vi "Unicode String to Integer [ ].vi"(0 "Char U16 [ ] IN":u16[](array[numeric]), 2 "From":enum16{"String", "U16 [ ]"}(ring), 7 "Unicode String":string, 11 "error in (no error)":errorcluster) -> (4 "Unicode String OUT":string, 8 "Char U16 [ ]":u16[](array[numeric]), 15 "error duplicate":errorcluster)   [LabVIEW 2020, in "Exaprom PDF.lvlib"]
doc: "Version 1.1\nDeveloped by Jean-Marc Simard\nCopyright © 2012, Exaprom Inc.\nAll rights reserved.\nLicense: BSD\n\nWith iTextSharp 4.1.6 (http://itextsharp.sourceforge.net)\nunder Mozilla Public License Version 1.1\n(http://www.mozilla.org/MPL/MPL-1.1.html)"
uses:
  <userlib>/labview-PDF-writer-master/Exaprom PDF.lvlib
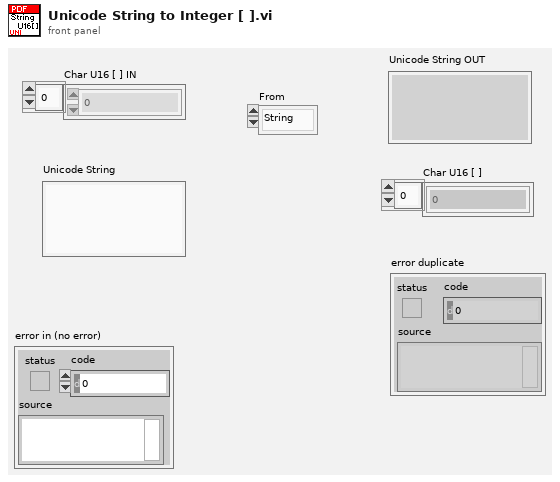
[diagram p1: front panel]
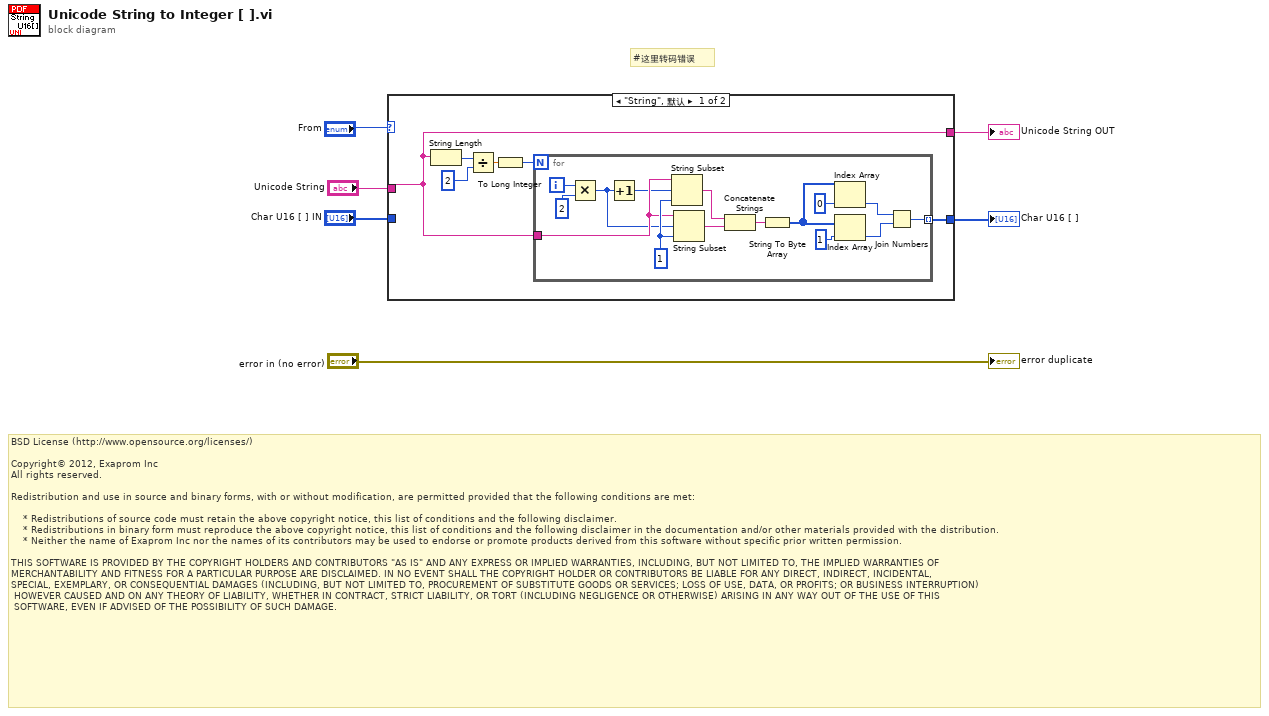
[diagram p0: block diagram]
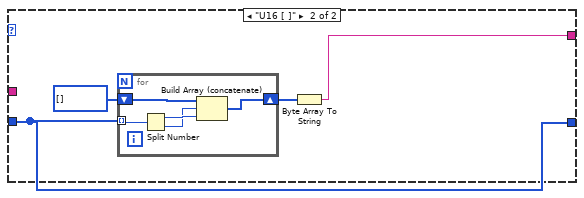
[diagram p2: hidden frame]
diagram:
  # "#这里转码错误"
  # "BSD License (http://www.opensource.org/licenses/)\n\nCopyright© 2012, Exaprom Inc\nAll rights reserved.\n\nRedistribution and use in source and binary forms, with or without modification, are permitted provided that the following conditions are met:\n\n    * Redistributions of source code must retain the above copyright notice, this list of conditions and the following disclaimer.\n    * Redistributions in binary form must reproduce the above copyright notice, this list of conditions and the following disclaimer in the documentation and/or other materials provided with the distribution.\n    * Neither the name of Exaprom Inc nor the names of its contributors may be used to endorse or promote products derived from this software without specific prior written permission.\n\nTHIS SOFTWARE IS PROVIDED BY THE COPYRIGHT HOLDERS AND CONTRIBUTORS \"AS IS\" AND ANY EXPRESS OR IMPLIED WARRANTIES, INCLUDING, BUT NOT LIMITED TO, THE IMPLIED WARRANTIES OF \nMERCHANTABILITY AND FITNESS FOR A PARTICULAR PURPOSE ARE DISCLAIMED. IN NO EVENT SHALL THE COPYRIGHT HOLDER OR CONTRIBUTORS BE LIABLE FOR ANY DIRECT, INDIRECT, INCIDENTAL,\nSPECIAL, EXEMPLARY, OR CONSEQUENTIAL DAMAGES (INCLUDING, BUT NOT LIMITED TO, PROCUREMENT OF SUBSTITUTE GOODS OR SERVICES; LOSS OF USE, DATA, OR PROFITS; OR BUSINESS INTERRUPTION)\n HOWEVER CAUSED AND ON ANY THEORY OF LIABILITY, WHETHER IN CONTRACT, STRICT LIABILITY, OR TORT (INCLUDING NEGLIGENCE OR OTHERWISE) ARISING IN ANY WAY OUT OF THE USE OF THIS\n SOFTWARE, EVEN IF ADVISED OF THE POSSIBILITY OF SUCH DAMAGE."
  n1 = case shown="\"String\", 默认" "From" {
    tunnel: "Unicode String" -> [w7 _]
    tunnel: [w12 w31] -> w4
    tunnel: "Char U16 [ ] IN" -> [_ w31]
    tunnel: [w7 w28] -> w1
    frame "String", Default {
      n2 = String Length(string=w7) -> (length=w9:i32)
      n3 = Divide(x=w9, y=2) -> (x/y=w8:dbl)
      n4 = To Long Integer(number=w8) -> (32bit integer=w11:i32)
      n5 = for {
        N: w11 -> [_]
        tunnel: w7 -> [w24]
        tunnel: [w13] -> w12 mode=indexing
        i -> [w27]
        w25 = 1 ("length (rest)")
        n6 = Multiply(x=w27, y=2) -> (x*y=w23:i32)
        n7 = Increment(x=w23) -> (x+1=w22:i32)
        n8 = String Subset(string=w24, offset (0)=w22, length (rest)=w25) -> (substring=w21:string)
        n9 = String Subset(string=w24, offset (0)=w23, length (rest)=w25) -> (substring=w20:string)
        n10 = Concatenate Strings(w21, w20) -> (w14:string)
        n11 = String To Byte Array(string=w14) -> (unsigned byte array=w17:u8[])
        n12 = Index Array(array=w17, index=0) -> (element=w18:u8)
        n13 = Index Array(array=w17, index=1) -> (element=w19:u8)
        n14 = Join Numbers(hi=w18, lo=w19) -> ((hi.lo)=w13:u16)
      }
    }
    frame "U16 [ ]" {
      n15 = for {
        tunnel: w31 -> [w36] mode=indexing
        shift-right: [w34] -> w29
        shift-left: u8[] [] -> [w35]
        n16 = Split Number(x=w36) -> (hi(x)=w33:u8, lo(x)=w32:u8)
        n17 = Build Array (concatenate)(w35, w32, w33) -> (w34:u8[])
      }
      n18 = Byte Array To String(unsigned byte array=w29) -> (string=w28:string)
    }
  }
  "Char U16 [ ]" <- w4
  "Unicode String OUT" <- w1
  "error duplicate" <- "error in (no error)"
